vi "CreateIntegerArray.vi"(11 "Array Inputs":T1) -> (2 "vector":dbl[](array[numeric]))   [LabVIEW 2015]
uses:
  <vilib>/imath/engines/lvmath2/RunTimeEngine/Managers/WorkSpace/UID Generator.vi
  <vilib>/imath/engines/lvmath2/RunTimeEngine/RunTimeType/NIMS_RunTimeType_From StrictType (excl LVString).vi
  <instcachedir>/0/NIMS_RunTimeType_From StrictType (excl LVString)_EB1C38A9BC5048DA9ABDA8F781E54D21.lvgen/NIMS_RunTimeType_From StrictType (excl LVString)_EB1C38A9BC5048DA9ABDA8F781E54D21_000.vi
  <vilib>/imath/engines/lvmath2/RunTimeEngine/LocalVariableDefStatement/MC_LocalVariableDefStatement_Display.vi
  <vilib>/imath/engines/lvmath2/RunTimeSupport/NIMS_Complex To Real.vi
  <instcachedir>/0/NIMS_Complex To Real_01315F44AA8B4CE79FEF95AE999DC25E.lvgen/NIMS_Complex To Real_01315F44AA8B4CE79FEF95AE999DC25E_001.vi
  <vilib>/imath/engines/lvmath2/RunTimeEngine/BuiltInFunctions/logramp/NIMS_logramp.vi
  <vilib>/imath/engines/lvmath2/RunTimeEngine/ErrorHandling/NIMS_Create Error From Enums.vi
  <vilib>/imath/engines/lvmath2/RunTimeEngine/BuiltInFunctions/linramp/NIMS_linramp.vi
  <vilib>/imath/engines/lvmath2/RunTimeEngine/Managers/SymbolTable/Clear UID.vi
  <vilib>/imath/engines/lvmath2/RunTimeEngine/NodeEndStatement/NIMS_NodeEndStatement_Output.vi
  <instcachedir>/0/NIMS_NodeEndStatement_Output_53EC0D466D134D7ABD903AC30B43404B.lvgen/NIMS_NodeEndStatement_Output_53EC0D466D134D7ABD903AC30B43404B_005.vi
  <vilib>/imath/engines/lvmath2/RunTimeEngine/ErrorHandling/NIMS_Finalize Error.vi
  <vilib>/imath/engines/lvmath2/RunTimeEngine/Managers/SymbolTable/NIMS_WorkSpace.lvlib
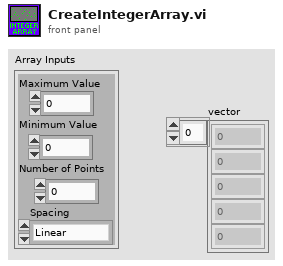
[diagram p1: front panel]
types:
  T1 = cluster{"Maximum Value":dbl, "Minimum Value":dbl, "Number of Points":dbl, "Spacing":enum16{"Linear", "Logarithmic"}}
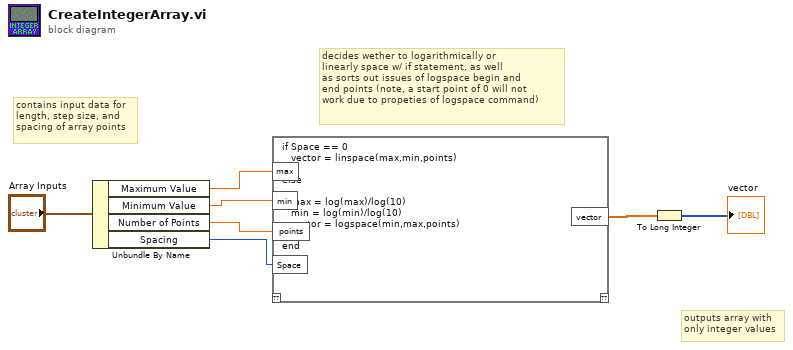
[diagram p0: block diagram]
diagram:
  # "outputs array with\nonly integer values"
  # "decides wether to logarithmically or\nlinearly space w/ if statement, as well\nas sorts out issues of logspace begin and\nend points (note, a start point of 0 will not\nwork due to propeties of logspace command)"
  # "contains input data for\nlength, step size, and \nspacing of array points"
  n1 = Unbundle By Name("Array Inputs") -> ("Maximum Value"=w6:dbl, "Minimum Value"=w5:dbl, "Number of Points"=w4:dbl, "Spacing"=w3:enum16{"Linear", "Logarithmic"})
  n2 = mathscript code="if Space == 0\n   vector = linspace(max,min,points)\n\nelse\n\n   max = log(max)/log(10)\n   min = log(min)/log(10)\n   vector = logspace(min,max,points)\n   \nend"("max"=w6, "min"=w5, "points"=w4, "Space"=w3) -> ("vector"=w2:dbl[])  [unwired: 1 in, 1 out]
  n3 = To Long Integer(number=w2) -> (32bit integer=→"vector":i32[])
